vi "Temperature.vi"() -> ()   [LabVIEW 2009, in "Magnet.lvclass"]
uses:
  Magnet.lvclass
panel:
  in  "old tempplot cluster":cluster{"time":dbl, "temp":dbl}
  out "start":dbl
  out "starttime":timestamp
  out "tempplot":cluster{"time":timestamp, "temp":dbl}[](array[cluster])
  in  "temparray":dbl[](array[numeric])
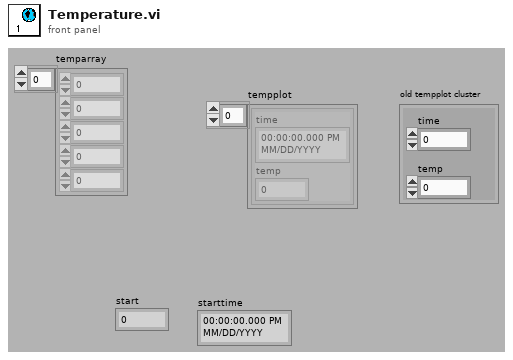
[diagram p1: front panel]
diagram:
